vi "RegisterWrite.vi"(7 "Write Data":T1 {"Register" format="%.0x"; "Slave Address" max=15 format="%.0x"}, 8 "error in (no error)":errorcluster, 9 "Number of Samples In":i32, 10 "Data Array":u8[][](array[numeric]), 11 "RFFE_Data":T2 {"Toggle (high to low)" items=["0", "1", "Z", "L", "H", "X", "T", "V"]; "X Array" items=["0", "1", "Z", "L", "H", "X", "T", "V"]; "Z Array" items=["0", "1", "Z", "L", "H", "X", "T", "V"]; "L Array" items=["0", "1", "Z", "L", "H", "X", "T", "V"]; "H Array" items=["0", "1", "Z", "L", "H", "X", "T", "V"]; "One Array" items=["0", "1", "Z", "L", "H", "X", "T", "V"]; "Zero Array" items=["0", "1", "Z", "L", "H", "X", "T", "V"]}) -> (0 "error out":errorcluster, 1 "Number of Samples Out":i32, 2 "Data Array Out":u8[][](array[numeric]), 3 "Configuratation Out":T2 {"Toggle (high to low)" items=["0", "1", "Z", "L", "H", "X", "T", "V"]; "X Array" items=["0", "1", "Z", "L", "H", "X", "T", "V"]; "Z Array" items=["0", "1", "Z", "L", "H", "X", "T", "V"]; "L Array" items=["0", "1", "Z", "L", "H", "X", "T", "V"]; "H Array" items=["0", "1", "Z", "L", "H", "X", "T", "V"]; "One Array" items=["0", "1", "Z", "L", "H", "X", "T", "V"]; "Zero Array" items=["0", "1", "Z", "L", "H", "X", "T", "V"]})   [LabVIEW 2013]
doc: "Builds MIPI RFFE Register Write with the specified data."
uses:
  Ctrls/RFFE_Data.ctl
  Ctrls/ClockDataChannels.ctl
  Ctrls/RegReadWrite.ctl
  Ctrls/Commands.ctl
  Ctrls/Read_Write_Data.ctl
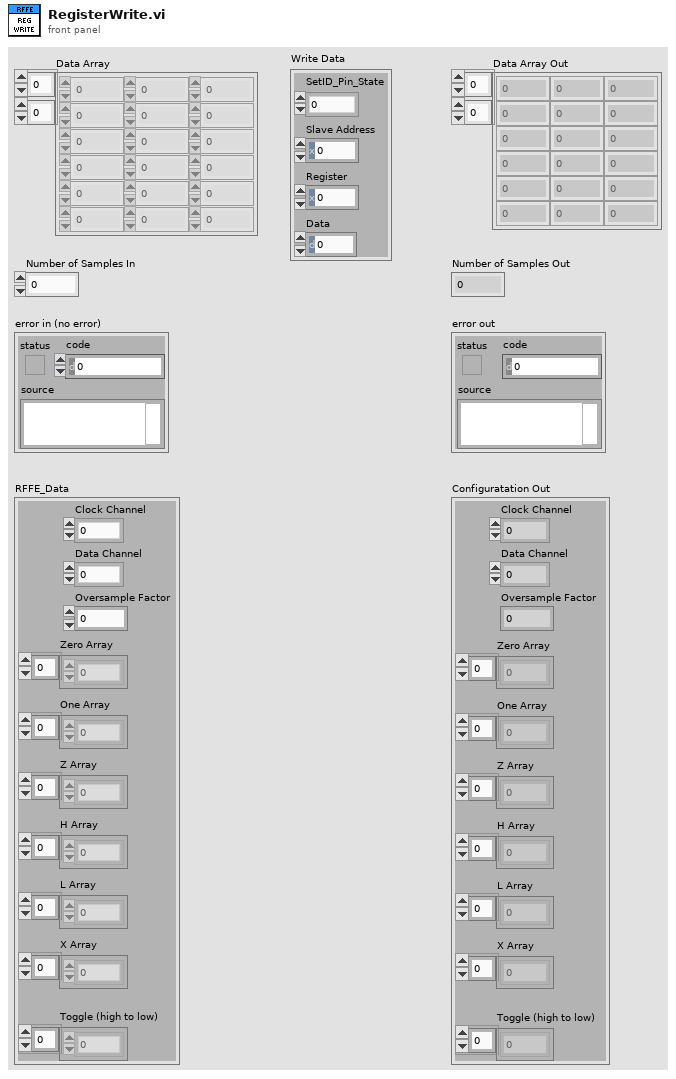
[diagram p1: front panel]
types:
  T1 = typedef "RegReadWrite.ctl" = cluster{"Slave Address":u8, "Register":u8, "Data":u8, "SetID_Pin_State":enum16{"0", "1", "Z"}}
  T2 = typedef "RFFE_Data.ctl" = cluster{"Clock Channel":T3, "Data Channel":T3, "Oversample Factor":u8, "Zero Array":u8[], "One Array":u8[], "Z Array ":u8[], "H Array":u8[], "L Array":u8[], "X Array":u8[], "Toggle (high to low)":u8[]}
  T3 = typedef "ClockDataChannels.ctl" = enum16{"0", "1"}
  T4 = typedef "Read_Write_Data.ctl" = cluster{"Data":u8, "Read/Write":enum16{"Read", "Write"}}
  T5 = typedef "Commands.ctl" = cluster{"Command":enum16{"Extended Register Write", "Extended Register Read", "Extended Register Write Long", "Extended Register Read Long", "Register Write", "Register Read", "Register 0 Write"}, "Data/Address/ByteCount":u8}
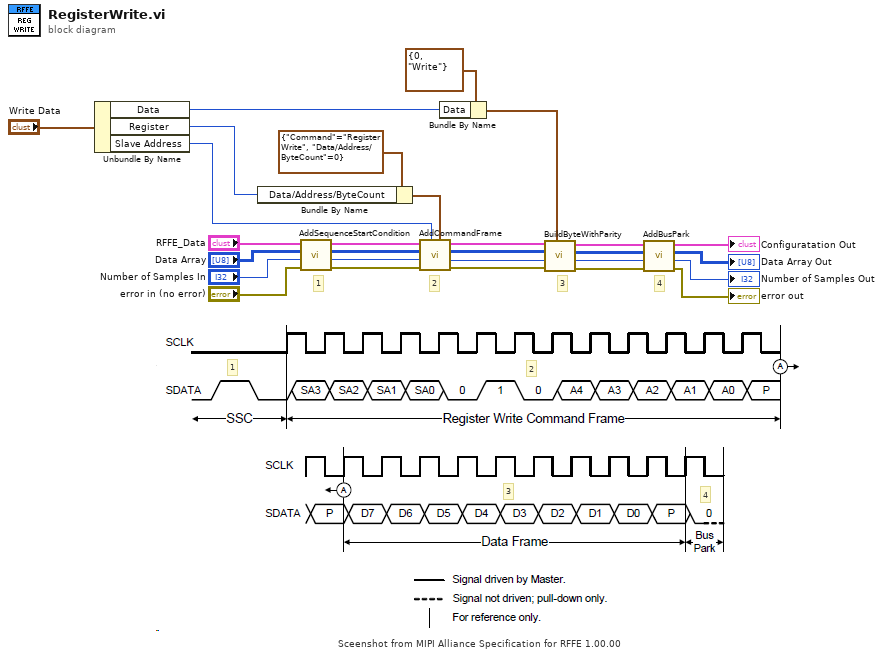
[diagram p0: block diagram]
diagram:
  # "Sceenshot from MIPI Alliance Specification for RFFE 1.00.00"
  # "4"
  # "3"
  # "2"
  # "1"
  # "4"
  # "3"
  # "2"
  # "1"
  n1 = Unbundle By Name("Write Data") -> ("Data"=w4:u8, "Register"=w14:u8, "Slave Address"=w1:u8)
  n2 = Bundle By Name(cluster=T5 {"Command"=enum."Register Write", "Data/Address/ByteCount"=0} ("Command"), "Data/Address/ByteCount"=w14) -> (w2:T5)
  n3 = call "AddSequenceStartCondition.vi"("error in (no error)"="error in (no error)", "Number of Samples In"="Number of Samples In", "Data Array In"="Data Array", "RFFE_Data In"="RFFE_Data") -> ("error out"=w18:errorcluster, "Number of Samples Out"=w26:i32, "Data Array Out"=w19:u8[][], "RFFE_Data Out"=w20:T2)  [unwired: 4 in]
  n4 = call "AddCommandFrame.vi"("Command"=w2, "Slave Address"=w1, "error in (no error)"=w18, "Number of Samples In"=w26, "Data Array In"=w19, "RFFE_Data"=w20) -> ("error out"=w21:errorcluster, "Number of Samples Out"=w23:i32, "Data Array Out"=w24:u8[][], "Configuratation Out"=w22:T2)  [unwired: 2 in]
  n5 = Bundle By Name(cluster=T4 {"Data"=0, "Read/Write"=enum."Write"} ("Read/Write Data"), "Data"=w4) -> (w3:T4)
  n6 = call "BuildByteWithParity.vi"("Read/Write Data"=w3, "error in"=w21, "Number of Samples In"=w23, "Data Array In"=w24, "RFFE_Data In"=w22) -> ("error out"=w13:errorcluster, "Number of Samples Out"=w11:i32, "Data Array Out"=w10:u8[][], "RFFE_Data Out"=w9:T2)  [unwired: 2 in, 1 out]
  n7 = call "AddBusPark.vi"("error in (no error)"=w13, "Number of Samples In"=w11, "Data Array In"=w10, "RFFE_Data In"=w9) -> ("error out"=→"error out":errorcluster, "Number of Samples Out"=→"Number of Samples Out":i32, "Data Array Out"=→"Data Array Out":u8[][], "RFFE_Data Out"=→"Configuratation Out":T2)  [unwired: 4 in]
